vi "Get LabVIEW EXE Name.vi"() -> (2 "LabVIEW EXE Name":string)   [LabVIEW 2015, in "Reaper.lvclass"]
uses:
  Reaper.lvclass
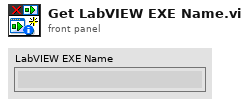
[diagram p1: front panel]
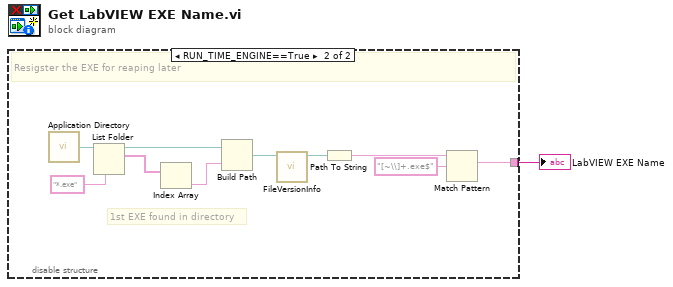
[diagram p0: block diagram]
diagram:
  n1 = disable-structure shown="RUN_TIME_ENGINE==True" {
    disable-tunnel: [_ w2] -> w1
    frame condition #0 (active) {
      # "Not an EXE -- Do nothing"
    }
    frame condition #1 {
      # "1st EXE found in directory"
      # "Resigster the EXE for reaping later"
      n2 = call <vilib>:"Application Directory.vi"() -> ("Application Directory"=w11:path)
      n3 = List Folder(path=w11, pattern="*.exe") -> (path out=w8:path, filenames=w9:string[])  [unwired: 2 in, 2 out]
      n4 = Index Array(array=w9) -> (element=w7:string)  [unwired: 1 in]
      n5 = Build Path(base path=w8, name or relative path=w7) -> (appended path=w6:path)
      n6 = call <vilib>:"FileVersionInfo.vi"("Application Path in"=w6) -> ("Application Path out"=w5:path)  [unwired: 7 in, 3 out]
      n7 = Path To String(path=w5) -> (string=w4:string)
      n8 = Match Pattern(string=w4, regular expression="[~\\]+.exe$") -> (match substring=w2:string)  [unwired: 1 in, 3 out]
    }
  }
  "LabVIEW EXE Name" <- w1
